vi "Find Template Base Name.vi"(8 "error in":errorcluster, 11 "source directory":path) -> (0 "error out":errorcluster, 3 "template base name":string)   [LabVIEW 2020, in "Template Tool.lvlib"]
uses:
  Template Tool.lvlib
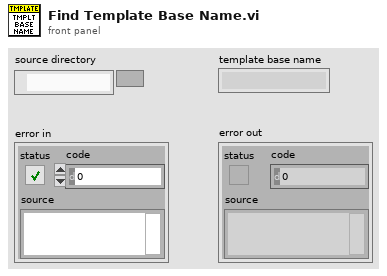
[diagram p1: front panel]
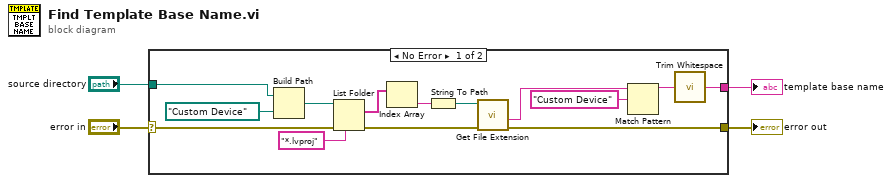
[diagram p0: block diagram]
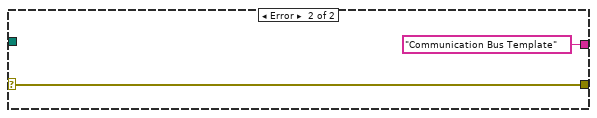
[diagram p2: hidden frame]
diagram:
  n1 = case shown="No Error" "error in" {
    selector: "error in" -> [w5 w20]
    tunnel: "source directory" -> [w9 _]
    tunnel: [w7 w20] -> w3
    tunnel: [w6 "Communication Bus Template" ("trimmed string")] -> w2
    frame No Error {
      n2 = Build Path(base path=w9, name or relative path=path "Custom Device") -> (appended path=w17:path)
      n3 = List Folder(path=w17, pattern="*.lvproj", error in=w5) -> (filenames=w15:string[], error out=w8:errorcluster)  [unwired: 1 in, 2 out]
      n4 = Index Array(array=w15) -> (element=w14:string)  [unwired: 1 in]
      n5 = String To Path(string=w14) -> (path=w13:path)
      n6 = call <vilib>:"Get File Extension.vi"("error in (no error)"=w8, "file"=w13) -> ("error out"=w7:errorcluster, "filename without extension"=w12:string)  [unwired: 5 in, 3 out]
      n7 = Match Pattern(string=w12, regular expression="Custom Device") -> (before substring=w10:string)  [unwired: 1 in, 3 out]
      n8 = call <vilib>:"Trim Whitespace.vi"("string"=w10) -> ("trimmed string"=w6:string)  [unwired: 1 in]
    }
    frame Error {
    }
  }
  "error out" <- w3
  "template base name" <- w2
